vi "read echarpe channel.vi"(8 "error in (no error)":errorcluster, 11 "Save Image ECHARPE in":refnum<class "Save Image ECHARPE.lvclass">) -> (0 "error out":errorcluster, 2 "echarpe channel":refnum<class "Channel ECHARPE.lvclass">, 3 "Save Image ECHARPE out":refnum<class "Save Image ECHARPE.lvclass">)   [LabVIEW 2018, in "Save Image ECHARPE.lvclass"]
uses:
  Save Image ECHARPE.lvclass
  C:/Users/Denis/Desktop/S4ACS/src/LabVIEW/Save Image/Save Image.lvclass
  S4ACS/src/LabVIEW/Channel ECHARPE/Channel ECHARPE.lvclass
  S4ACS/src/LabVIEW/Save Image/Save Image.lvclass
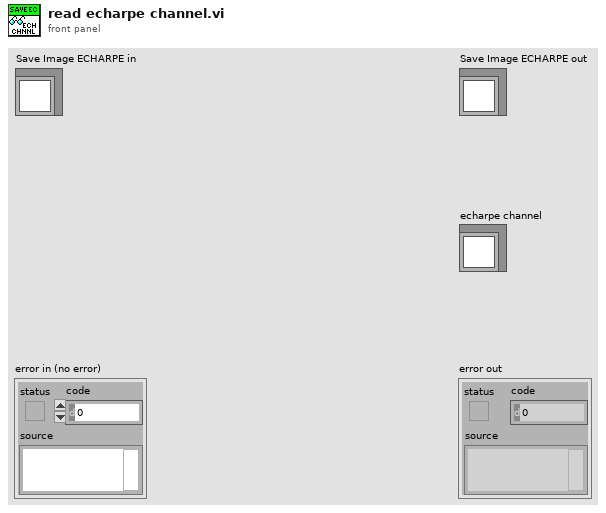
[diagram p1: front panel]
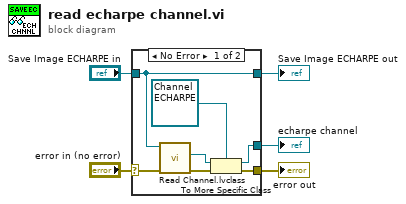
[diagram p0: block diagram]
diagram:
  n1 = case shown="No Error" "error in (no error)" {
    selector: "error in (no error)" -> [w9 w14]
    tunnel: [w8 w14] -> w4
    tunnel: [w10 w13] -> w2
    tunnel: "Save Image ECHARPE in" -> [w10 w13]
    tunnel: [w6 _] -> w1
    frame No Error {
      n2 = call "Read Channel.lvclass.vi"("error in (no error)"=w9, "Save Image in"=w10) -> ("error out"=w11:errorcluster, "Channel.lvclass"=w12:refnum<class "Channel.lvclass">)  [unwired: 7 in, 1 out]
      n3 = To More Specific Class(target class=refnum<class "Channel ECHARPE.lvclass"> refnum ("Channel ECHARPE.lvclass"), reference=w12, error in=w11) -> (specific class reference=w6:refnum<class "Channel ECHARPE.lvclass">, error out=w8:errorcluster)
    }
    frame Error {
    }
  }
  "error out" <- w4
  "Save Image ECHARPE out" <- w2
  "echarpe channel" <- w1
